vi "acquireValue.vi"(8 "error in (no error)":errorcluster, 10 "nextSample?":bool, 11 "closeShutter in":refnum<class "closeShutter.lvclass">) -> (0 "error out":errorcluster, 1 "function return":i32, 2 "variantData":variant, 3 "closeShutter out":refnum<class "closeShutter.lvclass">)   [LabVIEW 2016, in "SALLV_AtDome_Messaging.lvlib" / "closeShutter.lvclass"]
uses:
  closeShutter.lvclass
  ts_sallv_AtDome/SALLV_AtDome.lvlib
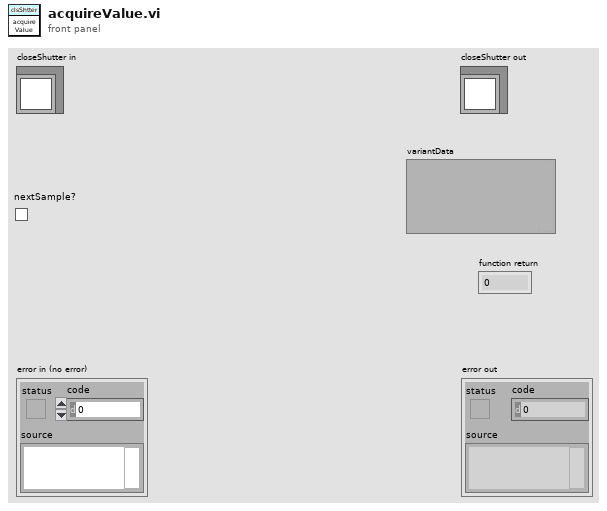
[diagram p1: front panel]
types:
  T1 = typedef "SALLV_AtDome.lvlib/command_closeShutter.ctl" = cluster{"close":bool}
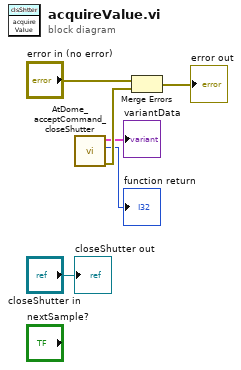
[diagram p0: block diagram]
diagram:
  n1 = call "AtDome_acceptCommand_closeShutter.vi"() -> ("error out"=w3:errorcluster, "function return"=→"function return":i32, "command_closeShutter_Ctl out"=→"variantData":T1)  [unwired: 9 in]
  n2 = Merge Errors("error in (no error)", w3) -> (→"error out":errorcluster)
  "closeShutter out" <- "closeShutter in"
